vi "TCP communication_target.vi"(7 "TCP command":T1(ring), 8 "error in":errorcluster, 10 "timeout ms":i32=25000, 11 "Data in":string[](array[string])) -> (0 "error out":errorcluster, 3 "Data out":string[](array[string]))   [LabVIEW 2011]
panel:
  in  "remote port":u16=6340
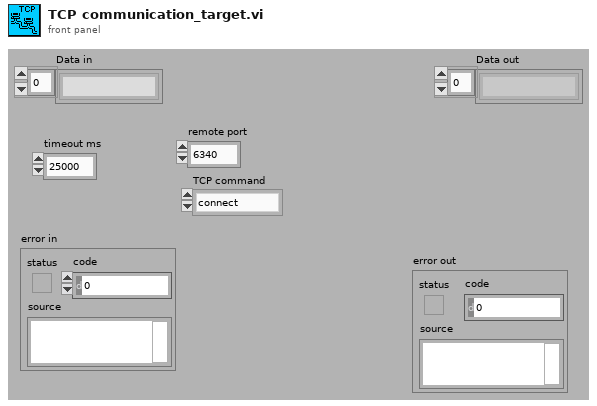
[diagram p1: front panel]
types:
  T1 = enum16{"connect", "receive data", "send data", "data transfer", "close"}
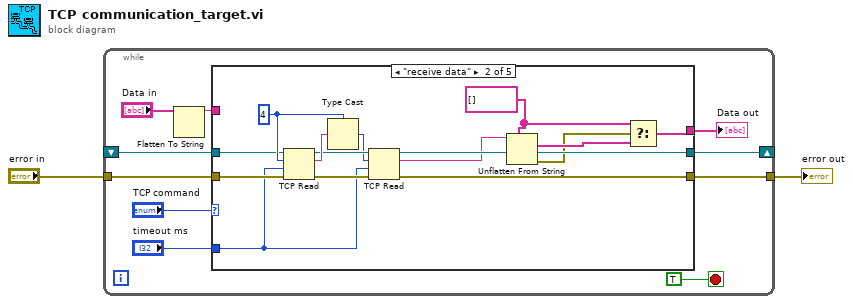
[diagram p0: block diagram]
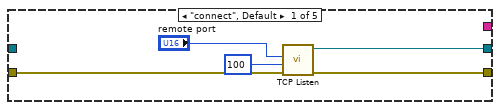
[diagram p2: hidden frame]
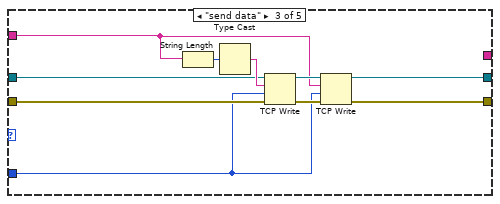
[diagram p3: hidden frame]
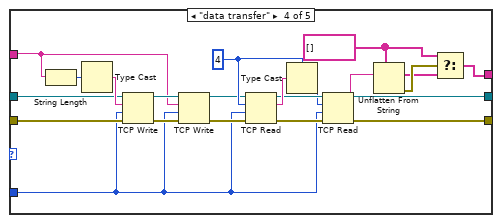
[diagram p4: hidden frame]
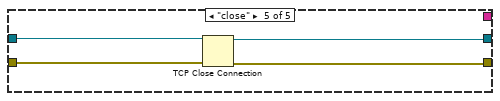
[diagram p5: hidden frame]
diagram:
  n1 = while {
    shift-right: [w12] -> _
    shift-left: _ -> [w10]
    tunnel: "error in" -> [w9]
    tunnel: [w8] -> w1
    stop <- TRUE stop-if-true
    n2 = Flatten To String(anything="Data in") -> (data string=w5:string)  [unwired: 3 in, 2 out]
    n3 = case shown="\"receive data\"" "TCP command" {
      tunnel: [w15 w26 w36 w50 w65] -> w12
      tunnel: w10 -> [_ w27 w37 w60 w66]
      tunnel: w9 -> [w13 w25 w34 w59 w68]
      tunnel: [w14 w22 w35 w47 w67] -> w8
      tunnel: [_ w18 _ w43 _] -> w4
      tunnel: w5 -> [_ _ w38 w58 _]
      tunnel: "timeout ms" -> [_ w23 w33 w48 _]
      frame "connect", Default {
        n4 = call <vilib>:"TCP Listen.vi"("error in (no error)"=w13, "timeout ms (wait forever: -1)"=100 ("timeout ms (60000)"), "port"="remote port") -> ("error out"=w14:errorcluster, "connection ID"=w15:refnum<k5>)  [unwired: 4 in, 3 out]
      }
      frame "receive data" {
        w20 = string[] [] ("Data In")
        w28 = 4
        n5 = TCP Read(connection ID=w27, bytes to read=w28, error in (no error)=w25, 9:w23) -> (connection ID out=w31:refnum<k5>, data out=w32:string, error out=w30:errorcluster)  [unwired: 1 in]
        n6 = Type Cast(type=w28, x=w32) -> (*(type *) &x=w29:i32)
        n7 = TCP Read(connection ID=w31, bytes to read=w29, error in (no error)=w30, 9:w23) -> (connection ID out=w26:refnum<k5>, data out=w24:string, error out=w22:errorcluster)  [unwired: 1 in]
        n8 = Unflatten From String(type=w20, binary string=w24) -> (value=w21:string[], error out=w19:errorcluster)  [unwired: 3 in, 1 out]
        n9 = Select(t=w20, s=w19, f=w21) -> (s? t:f=w18:string[])
      }
      frame "send data" {
        n10 = String Length(string=w38) -> (length=w40:i32)
        n11 = Type Cast(x=w40) -> (*(type *) &x=w39:string)  [unwired: 1 in]
        n12 = TCP Write(connection ID=w37, data in=w39, error in (no error)=w34, 9:w33) -> (connection ID out=w42:refnum<k5>, error out=w41:errorcluster)  [unwired: 1 out]
        n13 = TCP Write(connection ID=w42, data in=w38, error in (no error)=w41, 9:w33) -> (connection ID out=w36:refnum<k5>, error out=w35:errorcluster)  [unwired: 1 out]
      }
      frame "data transfer" {
        w44 = string[] [] ("Data In")
        w53 = 4
        n14 = String Length(string=w58) -> (length=w62:i32)
        n15 = Type Cast(x=w62) -> (*(type *) &x=w61:string)  [unwired: 1 in]
        n16 = TCP Write(connection ID=w60, data in=w61, error in (no error)=w59, 9:w48) -> (connection ID out=w64:refnum<k5>, error out=w63:errorcluster)  [unwired: 1 out]
        n17 = TCP Write(connection ID=w64, data in=w58, error in (no error)=w63, 9:w48) -> (connection ID out=w52:refnum<k5>, error out=w51:errorcluster)  [unwired: 1 out]
        n18 = TCP Read(connection ID=w52, bytes to read=w53, error in (no error)=w51, 9:w48) -> (connection ID out=w56:refnum<k5>, data out=w57:string, error out=w55:errorcluster)  [unwired: 1 in]
        n19 = Type Cast(type=w53, x=w57) -> (*(type *) &x=w54:i32)
        n20 = TCP Read(connection ID=w56, bytes to read=w54, error in (no error)=w55, 9:w48) -> (connection ID out=w50:refnum<k5>, data out=w49:string, error out=w47:errorcluster)  [unwired: 1 in]
        n21 = Unflatten From String(type=w44, binary string=w49) -> (value=w45:string[], error out=w46:errorcluster)  [unwired: 3 in, 1 out]
        n22 = Select(t=w44, s=w46, f=w45) -> (s? t:f=w43:string[])
      }
      frame "close" {
        n23 = TCP Close Connection(connection ID=w66, error in (no error)=w68) -> (connection ID out=w65:refnum<k5>, error out=w67:errorcluster)  [unwired: 1 in]
      }
    }
    "Data out" <- w4
  }
  "error out" <- w1
